vi "自动测试类型1统计结果.vi"   [LabVIEW 2010]
uses:
  全局量/自动测试结果.vi
  全局量/试验配置信息.vi
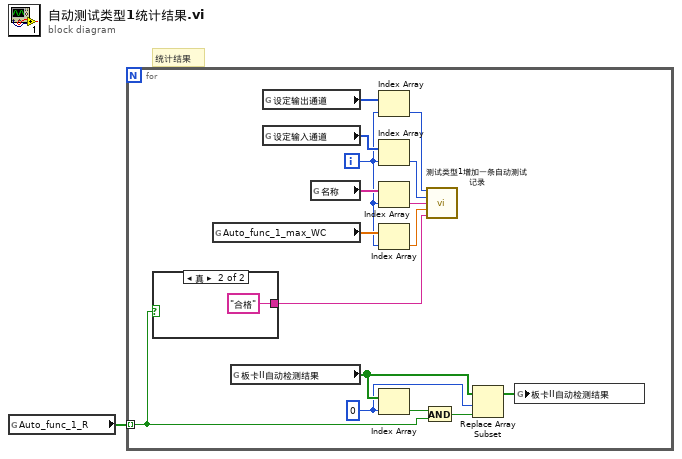
[diagram p0: block diagram]
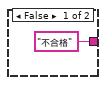
[diagram p2: hidden frame]
diagram:
  # "统计结果"
  n1 = global read "自动测试结果.vi" "Auto_func_1_R"() -> (w1:bool[])
  n2 = for {
    tunnel: w1 -> [w6] mode=indexing
    i -> [w3]
    w8 = 0 ("索引")
    n3 = case shown="真" w6 {
      tunnel: ["不合格" "合格"] -> w11
      frame False {
      }
      frame True {
      }
    }
    n4 = global read "自动测试结果.vi" "Auto_func_1_max_WC"() -> (w17:dbl[])
    n5 = global read "试验配置信息.vi" "板卡II自动检测结果"() -> (w9:bool[])
    n6 = global read "试验配置信息.vi" "设定输出通道"() -> (w16:u32[])
    n7 = global read "试验配置信息.vi" "设定输入通道"() -> (w15:u32[])
    n8 = global read "试验配置信息.vi" "名称"() -> (w4:string[])
    n9 = Index Array(array=w16, index=w3) -> (element=w14:u32)
    n10 = Index Array(array=w15, index=w3) -> (element=w13:u32)
    n11 = Index Array(array=w4, index=w3) -> (element=w2:string)
    n12 = Index Array(array=w17, index=w3) -> (element=w12:dbl)
    n13 = Index Array(array=w9, index=w8) -> (element=w7:bool)
    n14 = And(x=w7, y=w6) -> (x .and. y?=w5:bool)
    n15 = call "测试类型1增加一条自动测试记录.vi"("输出通道"=w14, "输入通道"=w13, "测试项"=w2, "最大误差"=w12, "测试结果"=w11) -> ()  [unwired: 11 in]
    n16 = Replace Array Subset(array=w9, new element=w5, index=w8) -> (w10:bool[])
    n17 = global write "试验配置信息.vi" "板卡II自动检测结果"(w10) -> ()
  }
